vi "Process.vi"(8 "error in":errorcluster, 11 "Logger":refnum<class "Logger.PGSQL.lvclass">) -> (0 "error out":errorcluster, 3 "Logger out":refnum<class "Logger.PGSQL.lvclass">)   [LabVIEW 2016, in "Logger.PGSQL.lvclass"]
doc: "---------------------------------------------------------------\nJKI State Machine Objects™\nhttp://jki.net/state-machine-objects/\nCopyright (C) 2005-2015, JKI <info@jki.net>\nALL RIGHTS RESERVED"
uses:
  <userlib>/LevyLab/Levylab Instruments/SMOs/Logger.PGSQL/Logger.PGSQL.lvclass
  C:/Program Files (x86)/National Instruments/LabVIEW 2016/vi.lib/JKI/JKI SMO/SMO/SMO.lvclass
  C:/Program Files (x86)/National Instruments/LabVIEW 2016/user.lib/LevyLab/Levylab Instruments/SMOs/Logger/Logger.lvclass
  <vilib>/JKI/JKI SMO/SMO/Typedefs/Parent Call--Enum.ctl
  <userlib>/LevyLab/postgreSQL/Data.PGSQL.lvclass
  <userlib>/LevyLab/Levylab Instruments/SMOs/Logger/Logger.lvclass
  <vilib>/JKI/JKI SMO/SMO/SMO.lvclass
panel:
  out "Data":variant
  out "Address":string
  # "For instructions on how to use the JKI State Machine Objects, examples and video tutorials, visit:\nhttp://jki.net/state-machine-objects/\n\nJKI State Machine Objects™\nhttp://jki.net/state-machine-objects/\nCopyright (C) 2005-2015, JKI <info@jki.net>\nALL RIGHTS RESERVED"
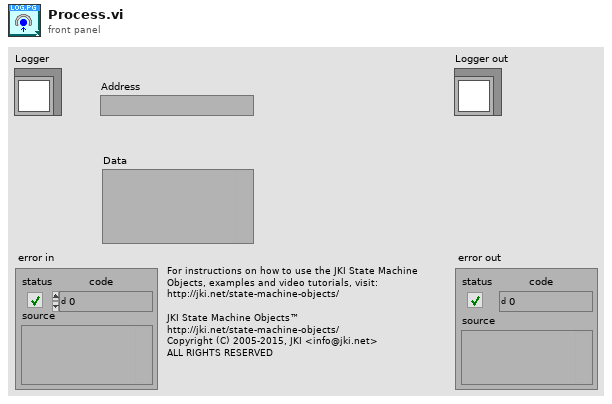
[diagram p1: front panel]
types:
  T1 = typedef "SMO.lvclass/Parent Call--Enum.ctl" = enum16{"Allows parent to run", "Does not request parent to run"}
  T2 = enum32{"invalid app kind", "Development System", "Run Time System", "Student Edition", "Embedded LabVIEW", "Evaluation", "Custom"}
  T3 = enum32{"Invalid", "Standard", "Closed", "Hidden", "Minimized", "Maximized"}
  T4 = enum32{"Bad", "Idle", "Run top level", "Running"}
  T5 = cluster{"Core":cluster{"Current VI Reference":refnum<vi>, "Close Panel on Exit?":bool, "error":errorcluster}, "Self Reference":refnum<class "Logger.PGSQL.lvclass">, "Data.PGSQL":refnum<class "Data.PGSQL.lvclass">, "variable address":string, "data in":variant, "data out":variant, "Debug Mode?":bool}
  T6 = cluster{"Current VI Reference":refnum<vi>, "Close Panel on Exit?":bool, "error":errorcluster}
  T7 = typedef "SMO.lvclass/Protected Events.ctl" = cluster{"StopProcesses":refnum<user-event>, "AbortProcesses":refnum<user-event>, "Config Changed":refnum<user-event>, "Dependency":refnum<user-event>}
  T8 = typedef "Logger.PGSQL.lvclass/PrivateEvents--Cluster.ctl" = cluster{"Set Address":refnum<user-event>, "Write Variable":refnum<user-event>}
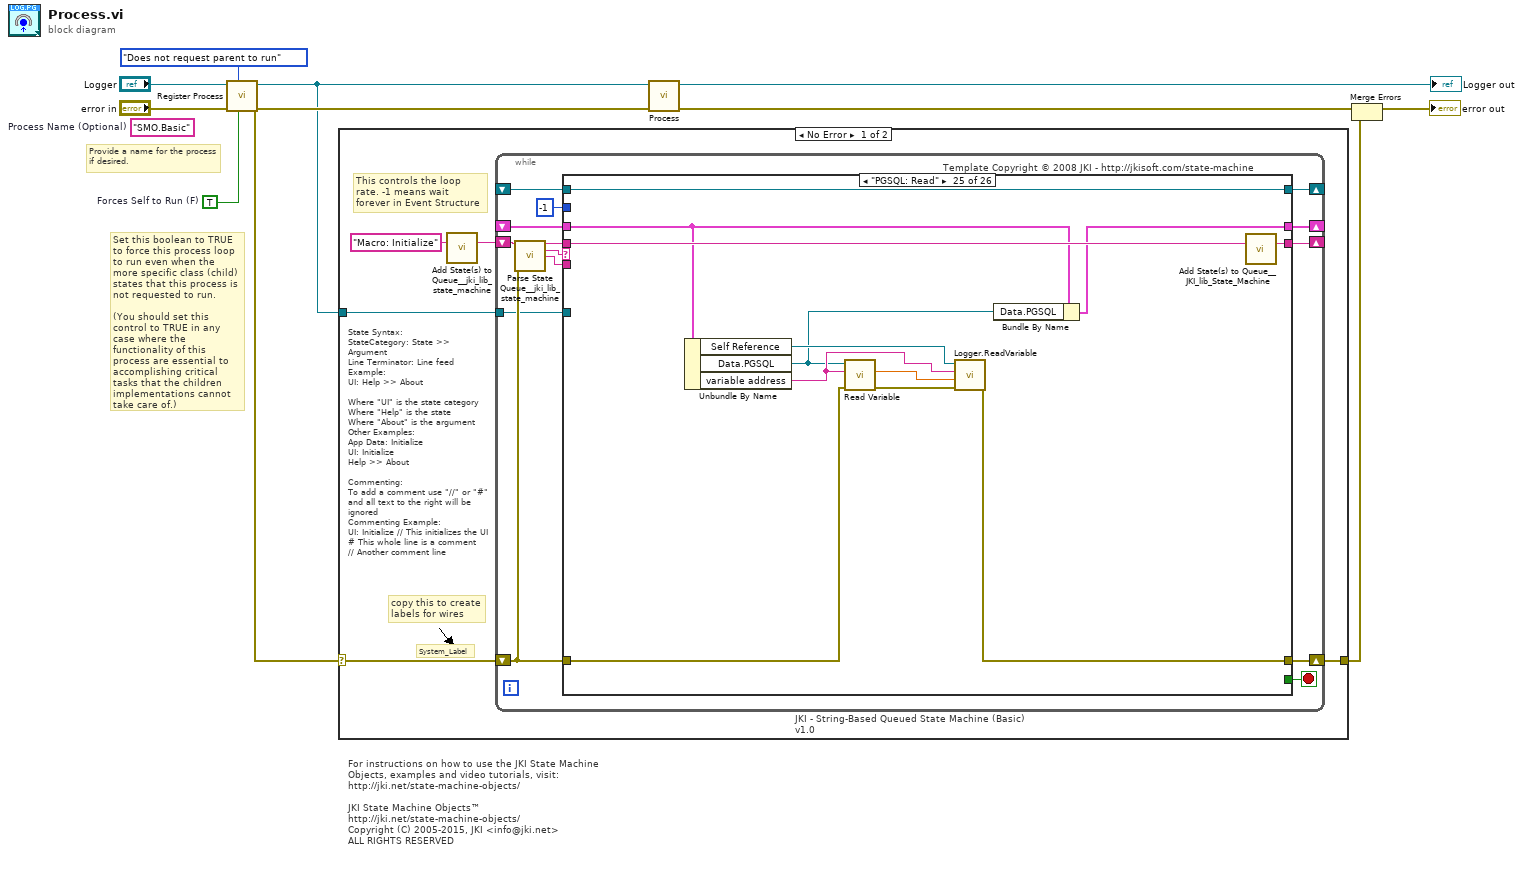
[diagram p0: block diagram]
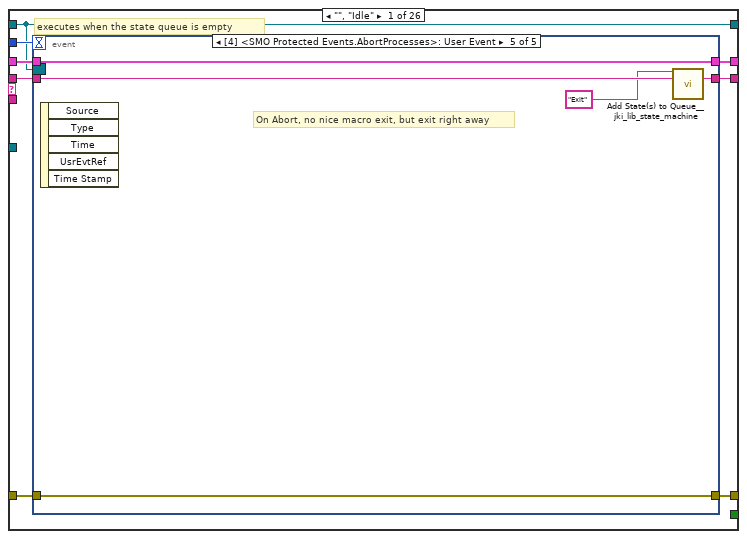
[diagram p2: hidden frame]
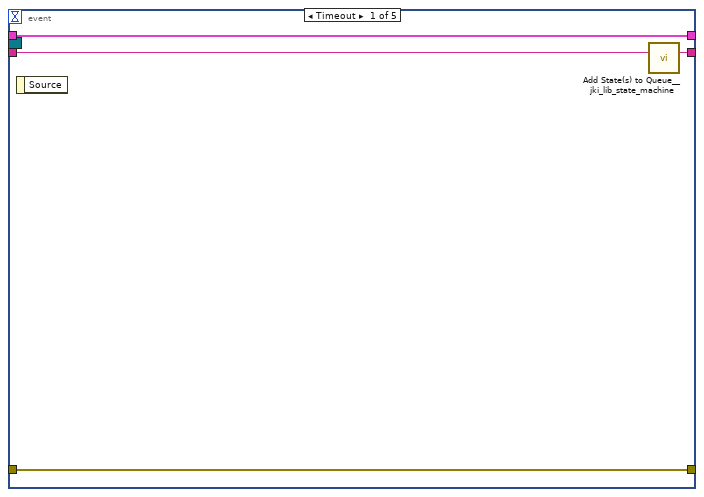
[diagram p3: hidden frame]
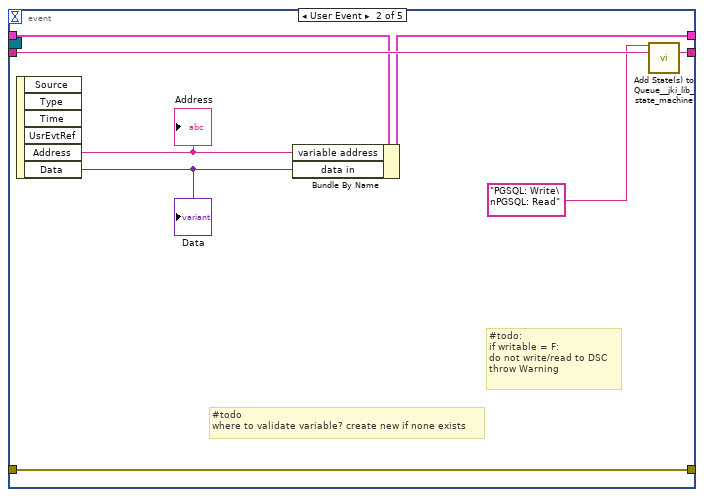
[diagram p4: hidden frame]
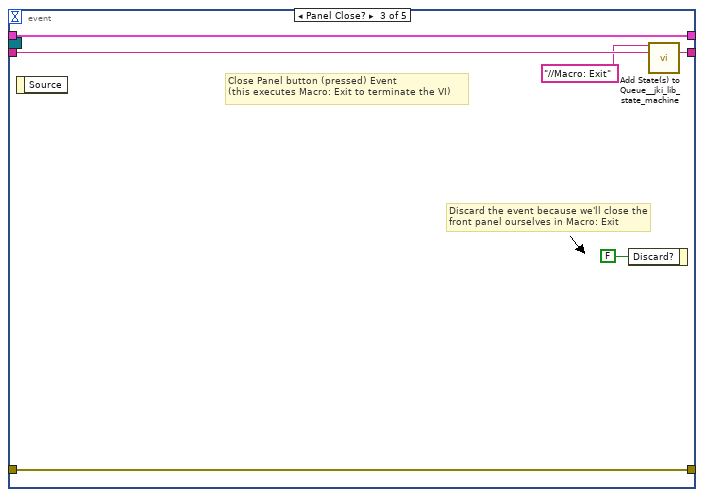
[diagram p5: hidden frame]
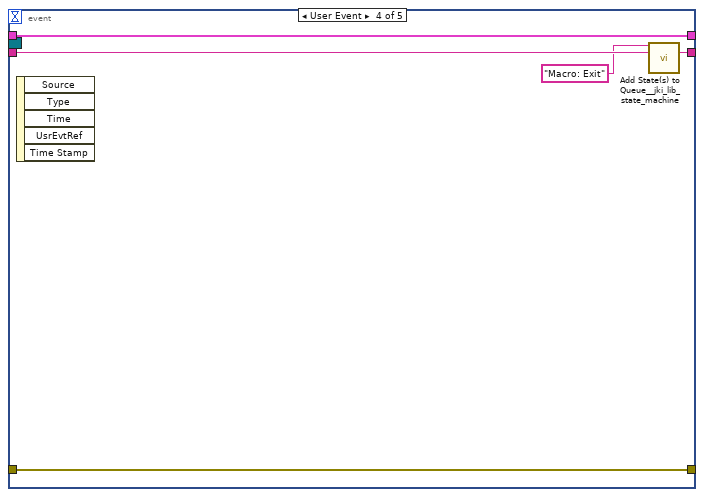
[diagram p6: hidden frame]
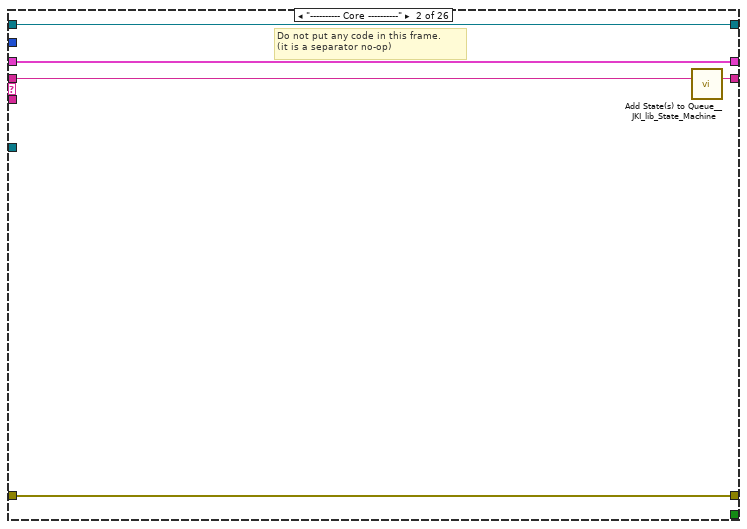
[diagram p7: hidden frame]
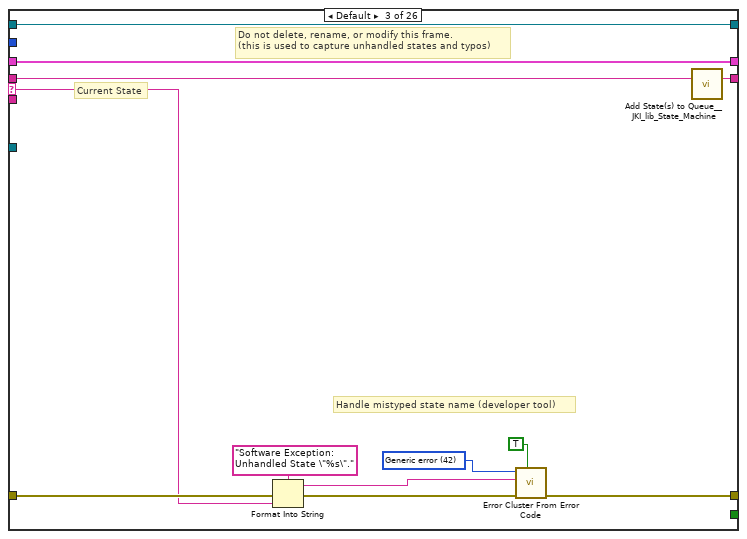
[diagram p8: hidden frame]
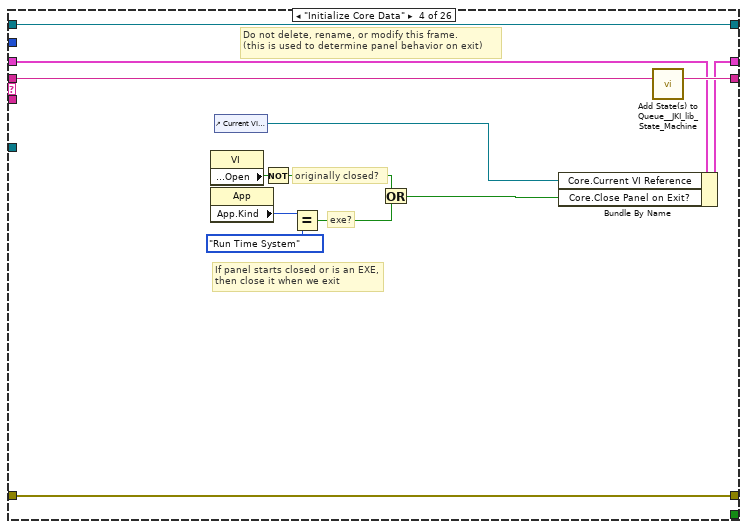
[diagram p9: hidden frame]
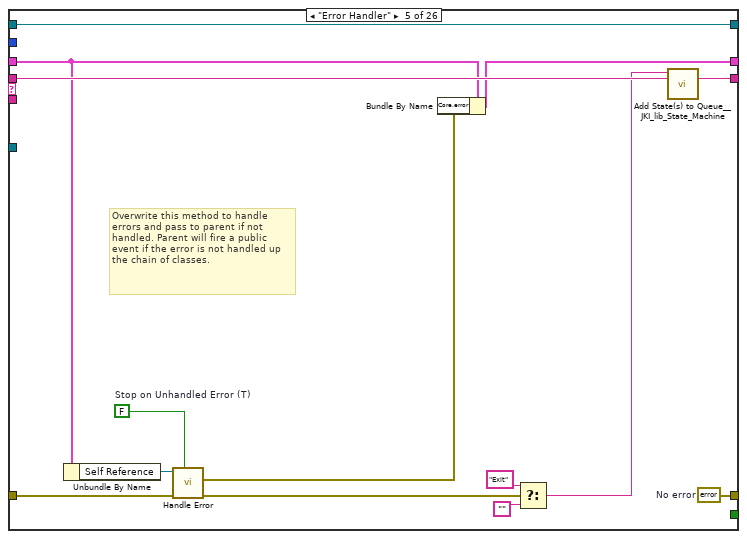
[diagram p10: hidden frame]
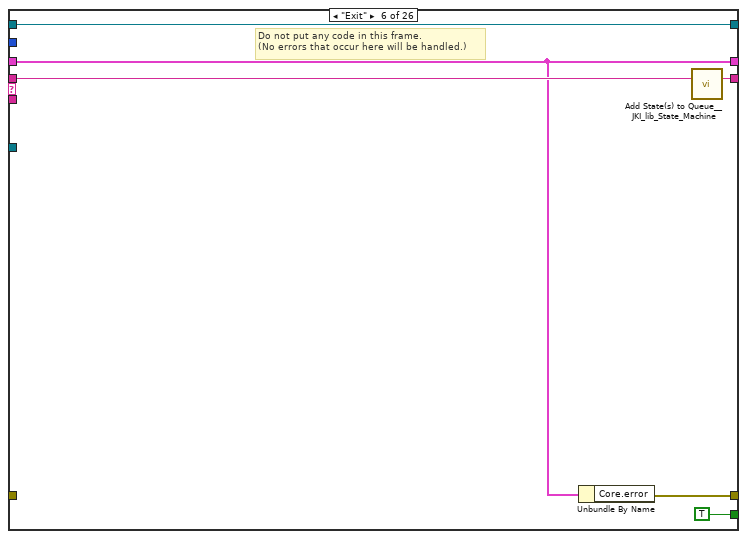
[diagram p11: hidden frame]
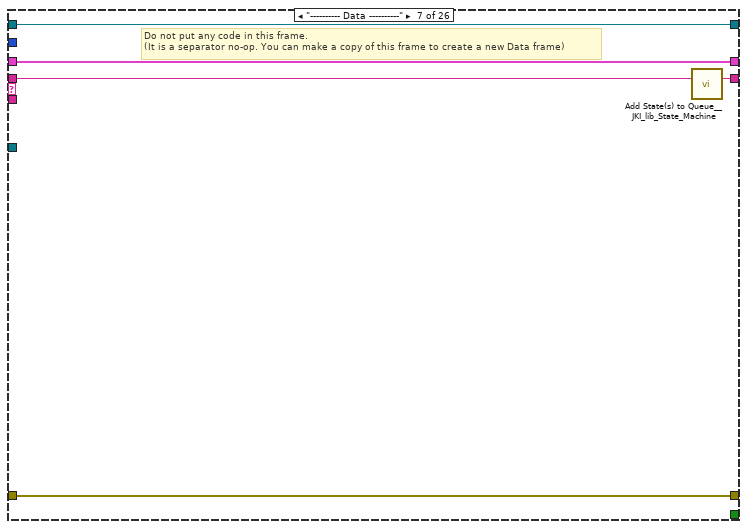
[diagram p12: hidden frame]
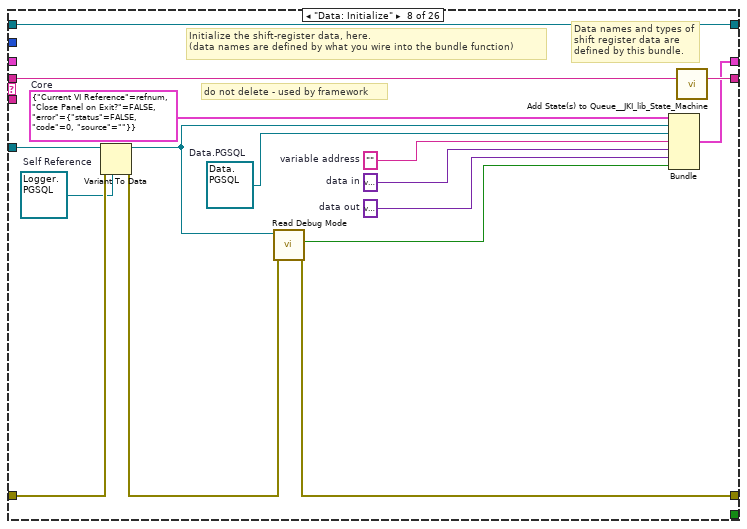
[diagram p13: hidden frame]
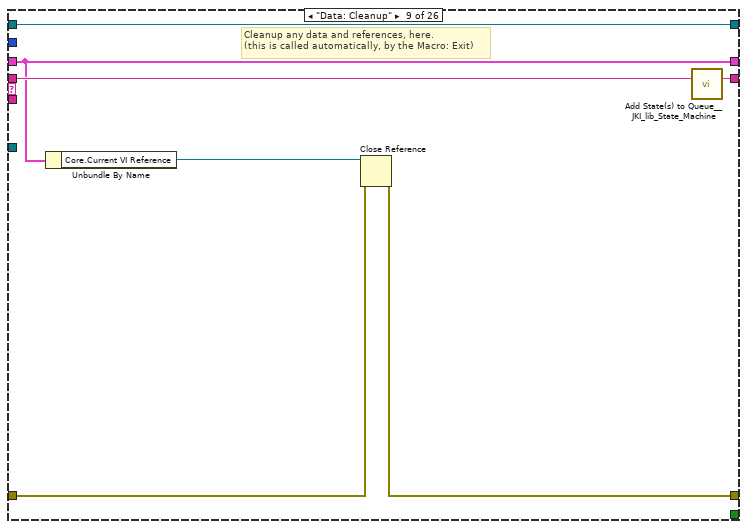
[diagram p14: hidden frame]
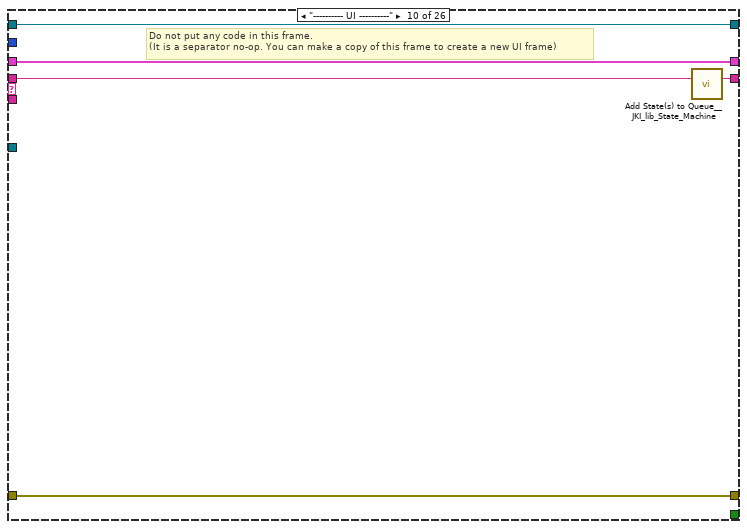
[diagram p15: hidden frame]
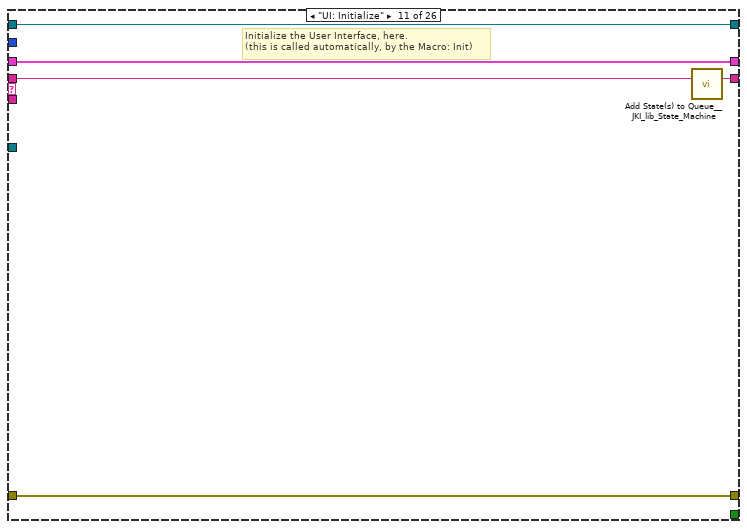
[diagram p16: hidden frame]
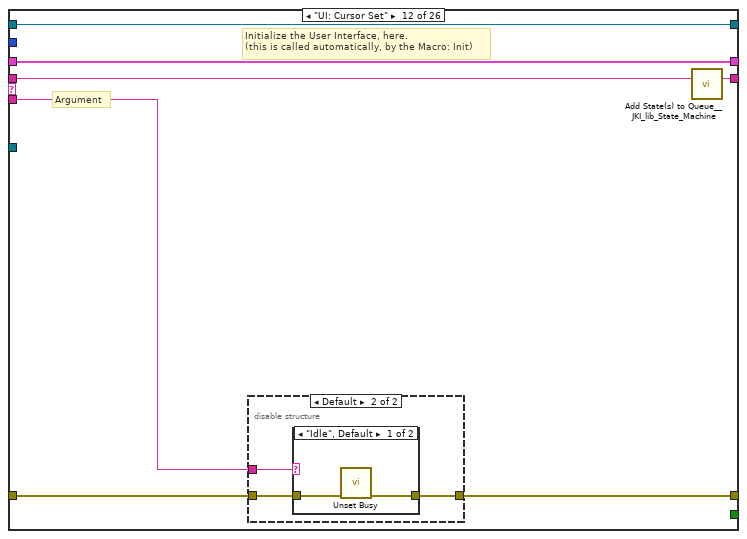
[diagram p17: hidden frame]
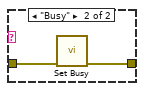
[diagram p19: hidden frame]
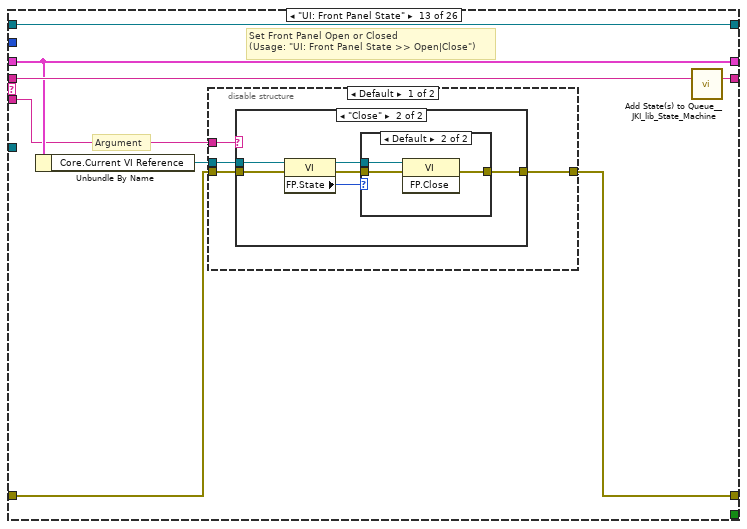
[diagram p20: hidden frame]
diagram:
  w1 = TRUE  # Forces Self to Run (F)
  (unwired) "SMO.Basic"  # Process Name (Optional)
  # "Provide a name for the process\nif desired."
  # "Set this boolean to TRUE to force this process loop to run even when the more specific class (child) states that this process is not requested to run.\n\n(You should set this control to TRUE in any case where the functionality of this process are essential to accomplishing critical tasks that the children implementations cannot take care of.)"
  # "For instructions on how to use the JKI State Machine Objects, examples and video tutorials, visit:\nhttp://jki.net/state-machine-objects/\n\nJKI State Machine Objects™\nhttp://jki.net/state-machine-objects/\nCopyright (C) 2005-2015, JKI <info@jki.net>\nALL RIGHTS RESERVED"
  n1 = call <vilib>:"Register Process.vi"("Forces Self to Run (F)"=w1, "Parent Call"=Parent_Call--Enum."Does not request parent to run", "error in (no error)"="error in", "SMO"="Logger") -> ("error out"=w7:errorcluster, "SMO out"=w6:refnum<class "Logger.PGSQL.lvclass">)  [unwired: 6 in]
  n2 = case shown="No Error" w7 {
    selector: w7 -> [w12 w340]
    tunnel: w6 -> [w13 _]
    tunnel: [w11 w340] -> w3
    frame No Error {
      # "State Syntax:\nStateCategory: State >> Argument\nLine Terminator: Line feed\nExample:\nUI: Help >> About\n\nWhere \"UI\" is the state category\nWhere \"Help\" is the state\nWhere \"About\" is the argument\nOther Examples:\nApp Data: Initialize\nUI: Initialize\nHelp >> About\n\nCommenting:\nTo add a comment use \"//\" or \"#\" and all text to the right will be ignored\nCommenting Example:\nUI: Initialize // This initializes the UI\n# This whole line is a comment\n// Another comment line"
      # "copy this to create labels for wires"
      # "This controls the loop rate. -1 means wait forever in Event Structure"
      # "System_Label"
      n3 = call <vilib>:"Add State(s) to Queue__jki_lib_state_machine.vi"("State(s) in (\"\")"="Macro: Initialize") -> ("States Out"=w15:string)  [unwired: 14 in]
      n4 = while "JKI - String-Based Queued State Machine (Basic) v1.0" {
        shift-right: [w22] -> _
        shift-left: _ -> [w21]
        shift-right: [w25] -> w11
        shift-left: w12 -> [w19]
        shift-right: [w24] -> _
        shift-left: w15 -> [w26]
        tunnel: w13 -> [w18]
        shift-right: [w17] -> _
        shift-left: _ -> [w16]
        stop <- w23 stop-if-true
        # "Template Copyright © 2008 JKI - http://jkisoft.com/state-machine"
        n5 = call <vilib>:"Parse State Queue__jki_lib_state_machine.vi"("State Queue"=w26, "Error In (no error)"=w19) -> ("Remaining States"=w28:string, "Current State"=w29:string, "Arguments"=w27:string)  [unwired: 11 in]
        n6 = case shown="\"PGSQL: Read\"" w29 {
          selector: w29 -> [_ _ w72 _ _ _ _ _ _ _ _ _ _ _ _ _ _ _ _ _ _ _ _ _ _ _]
          tunnel: w28 -> [w37 w70 w76 w95 w109 w115 w120 w136 w143 w148 w153 w160 w176 w208 w231 w250 w255 w266 w271 w284 w290 w295 w307 w318 w330 w339]
          tunnel: w27 -> [_ _ _ _ _ _ _ _ _ _ _ w154 w170 _ _ _ _ _ _ _ _ _ _ _ _ _]
          tunnel: w21 -> [w35 w67 w74 w86 w103 w111 w117 _ w138 w145 w151 w158 w172 w205 w216 w242 w252 w263 w268 w282 w288 w293 w301 w309 w321 w334]
          tunnel: [w34 w68 w78 w92 w104 w110 w118 w125 w139 w146 w150 w155 w173 w206 w212 w248 w253 w257 w269 w277 w286 w291 w297 w312 w327 w331] -> w25
          tunnel: w19 -> [w33 w68 w77 w92 w105 _ w118 w133 w140 w146 w150 w156 w174 w206 w211 w248 w253 w258 w269 w278 w286 w291 w298 w313 w322 w332]
          tunnel: [w36 w69 w75 w94 w108 w114 w119 w135 w142 w147 w152 w159 w175 w207 w230 w249 w254 w265 w270 w283 w289 w294 w306 w317 w329 w338] -> w24
          tunnel: [_ _ _ _ _ TRUE _ _ _ _ _ _ _ _ _ _ _ _ _ _ _ _ _ _ _ _] -> w23
          tunnel: [w32 w67 w74 w93 w102 w111 w117 w134 w138 w145 w151 w158 w172 w205 w216 w242 w252 w263 w268 w282 w288 w293 w300 w308 w320 w333] -> w22
          tunnel: -1 ("Timeout") -> [w31 _ _ _ _ _ _ _ _ _ _ _ _ _ _ _ _ _ _ _ _ _ _ _ _ _]
          tunnel: w18 -> [_ _ _ _ _ _ _ w131 _ _ _ _ _ _ w210 _ _ _ _ _ _ _ _ _ _ _]
          tunnel: [w30 w66 w71 w83 w107 w112 w116 w130 w137 w144 w149 w157 w169 w204 w229 w243 w251 w264 w267 w281 w287 w292 w305 w316 w328 w337] -> w17
          tunnel: w16 -> [w30 w66 w71 w83 w107 w112 w116 w130 w137 w144 w149 w157 w169 w204 w229 w243 w251 w264 w267 _ w287 w292 w305 w316 w328 w337]
          frame "", "Idle" {
            # "executes when the state queue is empty"
            n7 = event shown="[4] <SMO Protected Events.AbortProcesses>: User Event" {
              selector: w30 -> [_ _ _ _ _]
              dyn-events: _ -> [_ _ _ _ _]
              timeout: w31 -> [_ _ _ _ _]
              tunnel: w37 -> [w41 w49 w55 w60 w65]
              tunnel: [w40 w48 w54 w59 w64] -> w36
              tunnel: w35 -> [w39 w46 w52 w57 w62]
              tunnel: [w38 w47 w53 w58 w63] -> w34
              tunnel: w33 -> [w38 w47 w53 w58 w63]
              tunnel: [w39 w45 w52 w57 w62] -> w32
              event Timeout {
                n8 = event-data() -> ()  [unwired: 1 in, 1 out]
                n9 = call <vilib>:"Add State(s) to Queue__jki_lib_state_machine.vi"("State(s) in (\"\")"=w41) -> ("States Out"=w40:string)  [unwired: 14 in]
              }
              event User Event {
                # "#todo:\nif writable = F:\ndo not write/read to DSC\nthrow Warning"
                # "#todo\nwhere to validate variable? create new if none exists"
                n10 = event-data() -> ("Address"=w42:string, "Data"=w43:variant)  [unwired: 1 in, 4 out]
                "Address" <- w42
                "Data" <- w43
                n11 = Bundle By Name(cluster=w46, "variable address"=w42, "data in"=w43) -> (w45:T5)
                n12 = call <vilib>:"Add State(s) to Queue__jki_lib_state_machine.vi"("State(s) in Front (\"\")"="PGSQL: Write\nPGSQL: Read" ("State(s) in Front (\"\")"), "State(s) in (\"\")"=w49) -> ("States Out"=w48:string)  [unwired: 13 in]
              }
              event Panel Close? {
                # "Discard the event because we'll close the front panel ourselves in Macro: Exit"
                # "Close Panel button (pressed) Event\n(this executes Macro: Exit to terminate the VI)"
                n13 = event-data() -> ()  [unwired: 1 in, 1 out]
                n14 = event-data("Discard?"=FALSE) -> ()  [unwired: 1 in, 1 out]
                n15 = call <vilib>:"Add State(s) to Queue__jki_lib_state_machine.vi"("State(s) in Front (\"\")"="//Macro: Exit", "State(s) in (\"\")"=w55) -> ("States Out"=w54:string)  [unwired: 13 in]
              }
              event User Event {
                n16 = event-data() -> ()  [unwired: 1 in, 5 out]
                n17 = call <vilib>:"Add State(s) to Queue__jki_lib_state_machine.vi"("State(s) in Front (\"\")"="Macro: Exit", "State(s) in (\"\")"=w60) -> ("States Out"=w59:string)  [unwired: 13 in]
              }
              event User Event {
                # "On Abort, no nice macro exit, but exit right away"
                n18 = event-data() -> ()  [unwired: 1 in, 5 out]
                n19 = call <vilib>:"Add State(s) to Queue__jki_lib_state_machine.vi"("State(s) in Front (\"\")"="Exit", "State(s) in (\"\")"=w65) -> ("States Out"=w64:string)  [unwired: 13 in]
              }
            }
          }
          frame "---------- Core ----------" {
            # "Do not put any code in this frame.\n(it is a separator no-op)"
            n20 = call <vilib>:"Add State(s) to Queue__JKI_lib_State_Machine.vi"("State(s) in (\"\")"=w70) -> ("States Out"=w69:string)  [unwired: 14 in]
          }
          frame Default {
            w81 = 42 items=["No error", "Argument error", "Memory is full", "Out of zone", "End of file", "File already open", "Generic file I/O error", "File not found", "File permission error", "Disk is full", "Duplicate path", "Too many files open", "System feature not enabled", "Resource file not found", "Cannot add resource", "Resource not found", "Image not found", "Image memory error", "Pen does not exist", "Config type invalid", "Config token not found", "Config parse error", "Config memory error", "Bad external code format", "Bad external code offset", "External code not present", "Null window", "Destroy window error", "Null menu", "Print aborted", "Bad print record", "Print driver error", "Windows error during printing", "Memory error during printing", "Print dialog error", "Generic print error", "Invalid device refnum", "Device not found", "Device parameter error", "Device unit error", "Cannot open device", "Device call aborted", "Generic error", "Cancelled by user", "Object ID too low", "Object ID too high", "Object not in heap", "Unknown heap", "Unknown object (invalid DefProc)", "Unknown object (DefProc not in table)", "Message out of range", "Invalid (null) method", "Unknown message", "Manager call not supported", "Bad address", "Network operation in progress", "Network operation timed out", "Connection is busy", "Network attribute not supported", "Network error", "Address in use", "System out of memory", "Connection aborted", "Connection refused", "Not connected", "Already connected", "Connection closed", "Initialization error (interapplication manager)", "Bad occurrence", "Wait on unbound occurrence handler", "Occurrence queue overflow", "Datalog type conflict", "Unused", "Unrecognized type (interapplication manager)", "Memory corrupt", "Failed to make temporary DLL", "Old CIN version", "Drag socket not found", "Failed to load drop-object", "Failed to register OLE object", "Failed to release OLE object", "Format specifier type mismatch", "Unknown format specifier", "Too few format specifiers", "Too many format specifiers", "Scan failed", "Newer CIN version", "Error converting to variant", "Runtime menu error", "Password tampered", "Variant attribute not found", "Incompatible variant data type", "Event data is not available", "Event Store is not present", "Occurrence is not found", "Event Queue is not created", "Event info is not available", "Refnum passed is NULL", "Error retrieving Class GUID", "Error retrieving CoClass GUID", "Error retrieving TypeLib GUID.", "Bad built application magic bytes.", "Specific driver is different from the specific driver associated with the Logical Name.", "There is no session opened to the class driver.", "Max Error", "MAX - Error with config objects", "MAX - Error loading configuration", "MAX - Group not supported"]
            # "Current State"
            # "Do not delete, rename, or modify this frame.\n(this is used to capture unhandled states and typos)"
            # "Handle mistyped state name (developer tool)"
            n21 = Format Into String(format string="Software Exception: Unhandled State \"%s\"." ("message"), error in=w77, w72) -> (resulting string=w80:string, error out=w79:errorcluster)  [unwired: 1 in]
            n22 = call <vilib>:"Error Cluster From Error Code.vi"("show call chain? (False)"=TRUE, "error in (no error)"=w79, "error message (\"\")"=w80, "error code (0)"=w81) -> ("error out"=w78:errorcluster)  [unwired: 5 in]
            n23 = call <vilib>:"Add State(s) to Queue__JKI_lib_State_Machine.vi"("State(s) in (\"\")"=w76) -> ("States Out"=w75:string)  [unwired: 14 in]
          }
          frame "Initialize Core Data" {
            # "Do not delete, rename, or modify this frame.\n(this is used to determine panel behavior on exit)"
            # "originally closed?"
            # "exe?"
            # "If panel starts closed or is an EXE, then close it when we exit"
            n24 = property class="VI"() -> ("Front Panel.Open"=w91:bool)  [unwired: 2 in, 2 out]
            n25 = property class="App"() -> ("App.Kind"=w90:T2)  [unwired: 2 in, 2 out]
            n26 = control-ref of="Current VI Reference"() -> (w84:refnum<vi>)
            n27 = Not(x=w91) -> (.not. x?=w88:bool)
            n28 = Equal?(x=w90, y=T2."Run Time System" ("Application:Kind")) -> (x = y?=w87:bool)
            n29 = Or(x=w88, y=w87) -> (x .or. y?=w85:bool)
            n30 = Bundle By Name(cluster=w86, "Core.Current VI Reference"=w84, "Core.Close Panel on Exit?"=w85) -> (w93:T5)
            n31 = call <vilib>:"Add State(s) to Queue__JKI_lib_State_Machine.vi"("State(s) in (\"\")"=w95) -> ("States Out"=w94:string)  [unwired: 14 in]
          }
          frame "Error Handler" {
            w96 = FALSE  # Stop on Unhandled Error (T)
            w104 = errorcluster {"status"=FALSE, "code"=0, "source"=""}  # No error
            # "Overwrite this method to handle errors and pass to parent if not handled. Parent will fire a public event if the error is not handled up the chain of classes."
            n32 = Unbundle By Name(w103) -> ("Self Reference"=w106:refnum<class "Logger.PGSQL.lvclass">)
            n33 = call-dynamic "Handle Error.vi"("Stop on Unhandled Error (T)"=w96, "error in"=w105, "LevyLab"=w106) -> ("handling error"=w97:errorcluster, "Unhandled error"=w100:errorcluster)  [unwired: 6 in, 1 out]
            n34 = Bundle By Name(cluster=w103, "Core.error"=w100) -> (w102:T5)
            n35 = Select(t="Exit", s=w97, f="") -> (s? t:f=w101:string)
            n36 = call <vilib>:"Add State(s) to Queue__JKI_lib_State_Machine.vi"("State(s) in Front (\"\")"=w101, "State(s) in (\"\")"=w109) -> ("States Out"=w108:string)  [unwired: 13 in]
          }
          frame "Exit" {
            # "Do not put any code in this frame.\n(No errors that occur here will be handled.)"
            n37 = Unbundle By Name(w111) -> ("Core.error"=w110:errorcluster)
            n38 = call <vilib>:"Add State(s) to Queue__JKI_lib_State_Machine.vi"("State(s) in (\"\")"=w115) -> ("States Out"=w114:string)  [unwired: 14 in]
          }
          frame "---------- Data ----------" {
            # "Do not put any code in this frame.\n(It is a separator no-op. You can make a copy of this frame to create a new Data frame)"
            n39 = call <vilib>:"Add State(s) to Queue__JKI_lib_State_Machine.vi"("State(s) in (\"\")"=w120) -> ("States Out"=w119:string)  [unwired: 14 in]
          }
          frame "Data: Initialize" {
            w121 = refnum<class "Data.PGSQL.lvclass"> refnum  # Data.PGSQL
            w122 = variant  # data out
            w127 = variant  # data in
            w128 = ""  # variable address
            w129 = T6 {"Current VI Reference"=refnum, "Close Panel on Exit?"=FALSE, "error"={"status"=FALSE, "code"=0, "source"=""}}  # Core
            w132 = refnum<class "Logger.PGSQL.lvclass"> refnum  # Self Reference
            # "do not delete - used by framework"
            # "Data names and types of shift register data are defined by this bundle."
            # "Initialize the shift-register data, here.\n(data names are defined by what you wire into the bundle function)"
            n40 = Variant To Data(error in=w133, type=w132, Variant=w131) -> (data=w124:refnum<class "Logger.PGSQL.lvclass">, error out=w126:errorcluster)
            n41 = call <userlib>:"Read Debug Mode.vi"("error in (no error)"=w126, "Logger in"=w124) -> ("error out"=w125:errorcluster, "Debug Mode?"=w123:bool)  [unwired: 7 in, 1 out]
            n42 = Bundle("Core"=w129, "Self Reference"=w124, "Data.PGSQL"=w121, "variable address"=w128, "data in"=w127, "data out"=w122, "Debug Mode?"=w123) -> (w134:T5)  [unwired: 1 in]
            n43 = call <vilib>:"Add State(s) to Queue__JKI_lib_State_Machine.vi"("State(s) in (\"\")"=w136) -> ("States Out"=w135:string)  [unwired: 14 in]
          }
          frame "Data: Cleanup" {
            # "Cleanup any data and references, here.\n(this is called automatically, by the Macro: Exit)"
            n44 = Unbundle By Name(w138) -> ("Core.Current VI Reference"=w141:refnum<vi>)
            n45 = Close Reference(reference=w141, error in (no error)=w140) -> (error out=w139:errorcluster)
            n46 = call <vilib>:"Add State(s) to Queue__JKI_lib_State_Machine.vi"("State(s) in (\"\")"=w143) -> ("States Out"=w142:string)  [unwired: 14 in]
          }
          frame "---------- UI ----------" {
            # "Do not put any code in this frame.\n(It is a separator no-op. You can make a copy of this frame to create a new UI frame)"
            n47 = call <vilib>:"Add State(s) to Queue__JKI_lib_State_Machine.vi"("State(s) in (\"\")"=w148) -> ("States Out"=w147:string)  [unwired: 14 in]
          }
          frame "UI: Initialize" {
            # "Initialize the User Interface, here.\n(this is called automatically, by the Macro: Init)"
            n48 = call <vilib>:"Add State(s) to Queue__JKI_lib_State_Machine.vi"("State(s) in (\"\")"=w153) -> ("States Out"=w152:string)  [unwired: 14 in]
          }
          frame "UI: Cursor Set" {
            # "Argument"
            # "Initialize the User Interface, here.\n(this is called automatically, by the Macro: Init)"
            n49 = disable-structure shown="Default" {
              disable-tunnel: w156 -> [w161 w164]
              disable-tunnel: [w161 w163] -> w155
              disable-tunnel: w154 -> [_ w162]
              frame condition #0 {
              }
              frame condition #1 (active) {
                n50 = case shown="\"Idle\", Default" w162 {
                  tunnel: w164 -> [w166 w168]
                  tunnel: [w165 w167] -> w163
                  frame "Idle", Default {
                    n51 = call <vilib>:"Unset Busy.vi"("error in (no error)"=w166) -> ("error out"=w165:errorcluster)  [unwired: 10 in]
                  }
                  frame "Busy" {
                    n52 = call <vilib>:"Set Busy.vi"("error in (no error)"=w168) -> ("error out"=w167:errorcluster)  [unwired: 9 in, 1 out]
                  }
                }
              }
            }
            n53 = call <vilib>:"Add State(s) to Queue__JKI_lib_State_Machine.vi"("State(s) in (\"\")"=w160) -> ("States Out"=w159:string)  [unwired: 14 in]
          }
          frame "UI: Front Panel State" {
            # "Argument"
            # "Set Front Panel Open or Closed\n(Usage: \"UI: Front Panel State >> Open|Close\")"
            n54 = Unbundle By Name(w172) -> ("Core.Current VI Reference"=w171:refnum<vi>)
            n55 = disable-structure shown="Default" {
              disable-tunnel: w174 -> [w180 w203]
              disable-tunnel: [w179 w203] -> w173
              disable-tunnel: w171 -> [w178 _]
              disable-tunnel: w170 -> [w177 _]
              frame condition #0 (active) {
                n56 = case shown="\"Close\"" w177 {
                  tunnel: w180 -> [w184 w197]
                  tunnel: [w186 w198] -> w179
                  tunnel: w178 -> [w185 w195]
                  frame "Open", Default {
                    n57 = property class="VI"(reference=w185, error in=w184) -> (reference out=w182:refnum<vi>, error out=w183:errorcluster, "FP.State"=w181:T3)
                    n58 = case shown="\"Closed\"" w181 {
                      tunnel: [w189 w192] -> w186
                      tunnel: w183 -> [w188 w192]
                      tunnel: w182 -> [w187 _]
                      frame "Closed" {
                        n59 = invoke class="VI" method="FP.Open"(reference=w187, error in=w188, "Activate"=TRUE, "State"=T3."Standard") -> (error out=w189:errorcluster)  [unwired: 1 in, 4 out]
                      }
                      frame Default {
                      }
                    }
                  }
                  frame "Close" {
                    n60 = property class="VI"(reference=w195, error in=w197) -> (reference out=w194:refnum<vi>, error out=w196:errorcluster, "FP.State"=w193:T3)
                    n61 = case shown="Default" w193 {
                      tunnel: [w199 w202] -> w198
                      tunnel: w196 -> [w199 w201]
                      tunnel: w194 -> [_ w200]
                      frame "Invalid", "Closed" {
                      }
                      frame Default {
                        n62 = invoke class="VI" method="FP.Close"(reference=w200, error in=w201) -> (error out=w202:errorcluster)  [unwired: 1 in, 2 out]
                      }
                    }
                  }
                }
              }
              frame condition #1 {
              }
            }
            n63 = call <vilib>:"Add State(s) to Queue__JKI_lib_State_Machine.vi"("State(s) in (\"\")"=w176) -> ("States Out"=w175:string)  [unwired: 14 in]
          }
          frame "---------- Macro ----------" {
            # "Do not put any code in this frame.\n(It is a separator no-op. You can make a copy of this frame to create a new Macro frame)"
            n64 = call <vilib>:"Add State(s) to Queue__JKI_lib_State_Machine.vi"("State(s) in (\"\")"=w208) -> ("States Out"=w207:string)  [unwired: 14 in]
          }
          frame "Macro: Initialize" {
            w221 = "Process: Sync"
            # "This needs to be called here before Data: Initialize\nto ensure that the correct argument is present"
            # "Initialization Macro\n(This is called once, when the VI starts)"
            n65 = control-ref of="This VI"() -> (w223:refnum<vi>)
            n66 = property class="VI"(reference=w223) -> ("Exec.State"=w222:T4)  [unwired: 1 in, 2 out]
            n67 = call <userlib>:"Read Debug Mode.vi"("error in (no error)"=w211, "Logger in"=w210) -> ("error out"=w212:errorcluster, "Debug Mode?"=w209:bool)  [unwired: 7 in, 1 out]
            n68 = Equal?(x=w222, y=T4."Run top level") -> (x = y?=w227:bool)
            n69 = Select(t="Open", s=w209, f="Close") -> (s? t:f=w218:string)
            n70 = Select(t=w221, s=w227, f="") -> ()  [unwired: 1 out]
            n71 = call <vilib>:"Build State String with Arguments__JKI_lib_State_Machine.vi"("Arguments (\"\")"=w218, "State"="UI: Front Panel State") -> ("State with Arguments"=w215:string)  [unwired: 4 in]
            n72 = call <vilib>:"Add State(s) to Queue__JKI_lib_State_Machine.vi"("State(s) in Front (\"\")"="UI: Initialize", "State(s) in (\"\")"=w215) -> ("States Out"=w213:string)  [unwired: 13 in]
            n73 = call <vilib>:"Add State(s) to Queue__JKI_lib_State_Machine.vi"("State(s) in Front (\"\")"="Data: Initialize\nInitialize Core Data\nEvents: Register\nPGSQL: Open", "State(s) in (\"\")"=w221, "State(s) at Back (\"\")"=w213) -> ("States Out"=w224:string)  [unwired: 12 in]
            n74 = call <vilib>:"Add State(s) to Queue__JKI_lib_State_Machine.vi"("State(s) in Front (\"\")"=w224, "State(s) in (\"\")"=w231) -> ("States Out"=w230:string)  [unwired: 13 in]
          }
          frame "Macro: Exit" {
            # "Exit Macro\n(This is called once, when the VI exits)"
            n75 = Unbundle By Name(w242) -> ("Debug Mode?"=w233:bool, "Core.Close Panel on Exit?"=w247:bool)
            n76 = Select(t="Open", s=w233, f="Close") -> (s? t:f=w235:string)
            n77 = call <vilib>:"Build State String with Arguments__JKI_lib_State_Machine.vi"("Arguments (\"\")"=w235, "State"="UI: Front Panel State") -> ("State with Arguments"=w232:string)  [unwired: 4 in]
            n78 = Select(t=w232, s=w247, f="") -> (s? t:f=w245:string)
            n79 = call <vilib>:"Add State(s) to Queue__JKI_lib_State_Machine.vi"("State(s) in Front (\"\")"="PGSQL: Close\nData: Cleanup\nEvents: Unregister", "State(s) in (\"\")"="Process: Sync", "State(s) at Back (\"\")"="Exit") -> ("States Out"=w239:string)  [unwired: 12 in]
            n80 = call <vilib>:"Add State(s) to Queue__JKI_lib_State_Machine.vi"("State(s) in (\"\")"=w245, "State(s) at Back (\"\")"=w239) -> ("States Out"=w244:string)  [unwired: 13 in]
            n81 = call <vilib>:"Add State(s) to Queue__JKI_lib_State_Machine.vi"("State(s) in Front (\"\")"=w244, "State(s) in (\"\")"=w250) -> ("States Out"=w249:string)  [unwired: 13 in]
          }
          frame "---------- Process ----------" {
            # "Template Separator\n(You can make a copy of, or modify, this frame)"
            n82 = call <vilib>:"Add State(s) to Queue__JKI_lib_State_Machine.vi"("State(s) in (\"\")"=w255) -> ("States Out"=w254:string)  [unwired: 14 in]
          }
          frame "Process: Sync" {
            n83 = Unbundle By Name(w263) -> ("Self Reference"=w259:refnum<class "Logger.PGSQL.lvclass">)
            n84 = call <vilib>:"WaitOnProcessSync.vi"("error in (no error)"=w258, "SMO"=w259) -> ("error out"=w257:errorcluster, "Don't run?"=w262:bool)  [unwired: 7 in, 1 out]
            n85 = Select(t="Data: Cleanup\nEvents: Unregister\nExit", s=w262, f="") -> (s? t:f=w256:string)
            n86 = call <vilib>:"Add State(s) to Queue__JKI_lib_State_Machine.vi"("State(s) in Front (\"\")"=w256, "State(s) in (\"\")"=w266) -> ("States Out"=w265:string)  [unwired: 13 in]
          }
          frame "---------- Events ----------" {
            # "Template Separator\n(You can make a copy of, or modify, this frame)"
            n87 = call <vilib>:"Add State(s) to Queue__JKI_lib_State_Machine.vi"("State(s) in (\"\")"=w271) -> ("States Out"=w270:string)  [unwired: 14 in]
          }
          frame "Events: Register" {
            # "Expand to add\nmore events"
            n88 = Unbundle By Name(w282) -> ("Self Reference"=w279:refnum<class "Logger.PGSQL.lvclass">)
            n89 = call <vilib>:"GetProtectedEvents.vi"("SMO"=w279) -> ("error out"=w275:errorcluster, "SMO Protected Events"=w280:T7, "SMO out"=w274:refnum<class "Logger.PGSQL.lvclass">)  [unwired: 8 in]
            n90 = call <userlib>:"Logger.GetPrivateEvents.vi"("Logger"=w274) -> ("error out"=w272:errorcluster, "Private Events"=w273:T8)  [unwired: 8 in, 1 out]
            n91 = register-events(w280, w273) -> (reference out=w281:refnum<event-registration>, error out=w276:errorcluster)  [unwired: 2 in]
            n92 = Merge Errors(w272, w278, w276, w275) -> (w277:errorcluster)
            n93 = call <vilib>:"Add State(s) to Queue__JKI_lib_State_Machine.vi"("State(s) in (\"\")"=w284) -> ("States Out"=w283:string)  [unwired: 14 in]
          }
          frame "Events: Unregister" {
            n94 = Unregister For Events(event registration refnum=w287, error in=w286) -> (error out=w285:errorcluster)
            n95 = call <vilib>:"Clear Errors.vi"("error in (no error)"=w285) -> ()  [unwired: 5 in, 2 out]
            n96 = call <vilib>:"Add State(s) to Queue__JKI_lib_State_Machine.vi"("State(s) in (\"\")"=w290) -> ("States Out"=w289:string)  [unwired: 14 in]
          }
          frame "---------- PGSQL ----------" {
            n97 = call <vilib>:"Add State(s) to Queue__JKI_lib_State_Machine.vi"("State(s) in (\"\")"=w295) -> ("States Out"=w294:string)  [unwired: 14 in]
          }
          frame "PGSQL: Open" {
            n98 = Unbundle By Name(w301) -> ("Data.PGSQL"=w304:refnum<class "Data.PGSQL.lvclass">)
            n99 = call <userlib>:"Set Connection Info.vi"("Data.PG in"=w304, "username"="example_inst" ("user"), "error in (no error)"=w298) -> ("Data.PG out"=w302:refnum<class "Data.PGSQL.lvclass">, "error out"=w303:errorcluster)  [unwired: 6 in]
            n100 = call-dynamic "Open.vi"("error in (no error)"=w303, "Data.PG in"=w302) -> ("error out"=w297:errorcluster, "Data.PG out"=w299:refnum<class "Data.PGSQL.lvclass">)  [unwired: 8 in]
            n101 = Bundle By Name(cluster=w301, "Data.PGSQL"=w299) -> (w300:T5)
            n102 = call <vilib>:"Add State(s) to Queue__JKI_lib_State_Machine.vi"("State(s) in (\"\")"=w307) -> ("States Out"=w306:string)  [unwired: 14 in]
          }
          frame "PGSQL: Write" {
            n103 = Unbundle By Name(w309) -> ("Data.PGSQL"=w311:refnum<class "Data.PGSQL.lvclass">, "variable address"=w315:string, "data in"=w314:variant)
            n104 = call <userlib>:"Write Variable.vi"("error in (no error)"=w313, "Data"=w314, "variable"=w315, "Data.PG in"=w311) -> ("error out"=w312:errorcluster, "Data.PG out"=w310:refnum<class "Data.PGSQL.lvclass">)  [unwired: 5 in, 1 out]
            n105 = Bundle By Name(cluster=w309, "Data.PGSQL"=w310) -> (w308:T5)
            n106 = call <vilib>:"Add State(s) to Queue__JKI_lib_State_Machine.vi"("State(s) in (\"\")"=w318) -> ("States Out"=w317:string)  [unwired: 14 in]
          }
          frame "PGSQL: Read" {
            n107 = Unbundle By Name(w321) -> ("Self Reference"=w326:refnum<class "Logger.PGSQL.lvclass">, "Data.PGSQL"=w319:refnum<class "Data.PGSQL.lvclass">, "variable address"=w324:string)
            n108 = call <userlib>:"Read Variable.vi"("error in (no error)"=w322, "PG path"=w324, "Data.PGQL in"=w319) -> ("error out"=w323:errorcluster, "Value"=w325:dbl)  [unwired: 4 in, 3 out]
            n109 = call <userlib>:"Logger.ReadVariable.vi"("error in (no error)"=w323, "Data"=w325, "Address"=w324, "Logger"=w326) -> ("error out"=w327:errorcluster)  [unwired: 6 in, 1 out]
            n110 = Bundle By Name(cluster=w321, "Data.PGSQL"=w319) -> (w320:T5)
            n111 = call <vilib>:"Add State(s) to Queue__JKI_lib_State_Machine.vi"("State(s) in (\"\")"=w330) -> ("States Out"=w329:string)  [unwired: 14 in]
          }
          frame "PGSQL: Close" {
            n112 = Unbundle By Name(w334) -> ("Data.PGSQL"=w336:refnum<class "Data.PGSQL.lvclass">)
            n113 = call-dynamic "Close.vi"("error in (no error)"=w332, "Data.PG in"=w336) -> ("error out"=w331:errorcluster, "Data.PG out"=w335:refnum<class "Data.PGSQL.lvclass">)  [unwired: 8 in]
            n114 = Bundle By Name(cluster=w334, "Data.PGSQL"=w335) -> (w333:T5)
            n115 = call <vilib>:"Add State(s) to Queue__JKI_lib_State_Machine.vi"("State(s) in (\"\")"=w339) -> ("States Out"=w338:string)  [unwired: 14 in]
          }
        }
      }
    }
    frame Error {
    }
  }
  n116 = call-parent "Process.vi"("error in"=w7, "Logger"=w6) -> ("error out"=w4:errorcluster, "Logger out"=→"Logger out":refnum<class "Logger.PGSQL.lvclass">)  [unwired: 8 in]
  n117 = Merge Errors(w4, w3) -> (→"error out":errorcluster)
